vi "Open OPC connections.vi"(8 "error in (no error)":errorcluster, 11 "OPC adressess":T2={"Data Received  URL"="opc:\\cyberlogic.opcserverDA\\UB.DataReceived", "Data Ready URL"="opc:\\cyberlogic.opcserverDA\\UB.DataReady", "Message URL"="opc:\\cyberlogic.opcserverDA\\UB.MagHistString"}) -> (0 "error IO":errorcluster, 3 "OPC connections":T1)   [LabVIEW 2015]
uses:
  OPC Adresses.ctl
  OPC connections.ctl
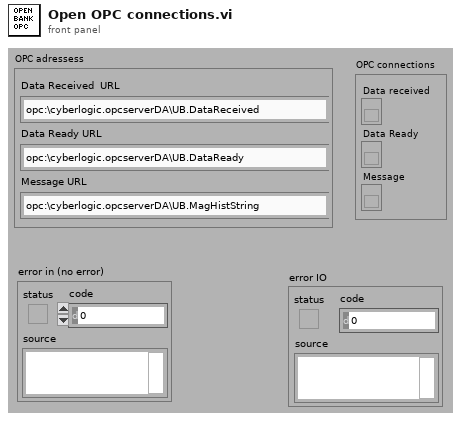
[diagram p1: front panel]
types:
  T1 = typedef "OPC connections.ctl" = cluster{"Data received":refnum<k13>, "Data Ready":refnum<k13>, "Message":refnum<k13>}
  T2 = typedef "OPC Adresses.ctl" = cluster{"Data Received  URL":string, "Data Ready URL":string, "Message URL":string}
  T3 = enum16{"Read", "Write", "ReadWrite", "BufferedRead", "BufferedReadWrite"}
  T4 = cluster{"connection id":refnum<k13>, "connection id":refnum<k13>, "connection id":refnum<k13>}
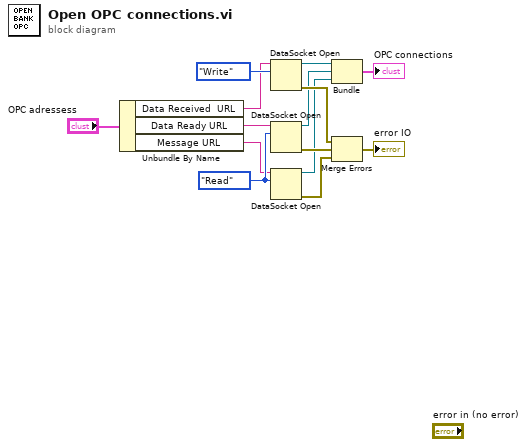
[diagram p0: block diagram]
diagram:
  w13 = T3."Read" ("mode")
  n1 = Unbundle By Name("OPC adressess") -> ("Data Received  URL"=w7:string, "Data Ready URL"=w6:string, "Message URL"=w5:string)
  n2 = DataSocket Open(10:T3."Write" ("mode"), 11:w7) -> (0:w14:errorcluster, 3:w4:refnum<k13>)  [unwired: 2 in]
  n3 = DataSocket Open(10:w13, 11:w6) -> (0:w9:errorcluster, 3:w3:refnum<k13>)  [unwired: 2 in]
  n4 = DataSocket Open(10:w13, 11:w5) -> (0:w11:errorcluster, 3:w2:refnum<k13>)  [unwired: 2 in]
  n5 = Bundle("connection id"=w4, "connection id"=w3, "connection id"=w2) -> (→"OPC connections":T4)  [unwired: 1 in]
  n6 = Merge Errors(w14, w9, w11) -> (→"error IO":errorcluster)
